vi "Save Globals.vi"(8 "error in (no error)":errorcluster, 10 "Prompt for Conflicts (T)":bool=TRUE, 11 "Engine in":refnum<class "Engine.lvclass">) -> (0 "error out":errorcluster, 3 "Engine out":refnum<class "Engine.lvclass">)   [LabVIEW 2020, in "TSnax.lvlib" / "Engine.lvclass"]
uses:
  Engine.lvclass
  Engine.lvclass/Engine.ctl
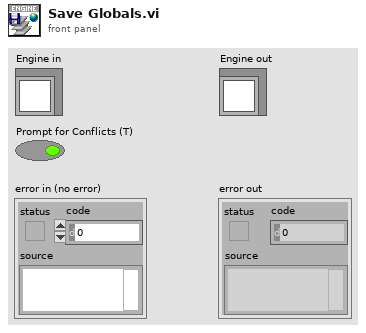
[diagram p1: front panel]
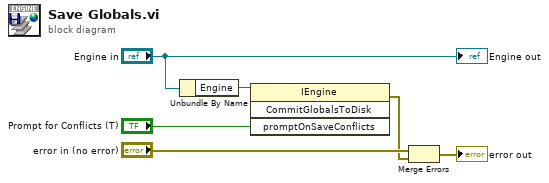
[diagram p0: block diagram]
diagram:
  n1 = Unbundle By Name("Engine in") -> ("Engine"=w4:refnum<k7>)
  n2 = invoke class="IEngine" method="CommitGlobalsToDisk"(reference=w4, "promptOnSaveConflicts"="Prompt for Conflicts (T)") -> (error out=w1:errorcluster)  [unwired: 2 in, 3 out]
  n3 = Merge Errors("error in (no error)", w1) -> (→"error out":errorcluster)
  "Engine out" <- "Engine in"
